vi "Gas Rack Main (FPGA).vi"() -> ()   [LabVIEW 2013]
uses:
  TypeDef/FPGADataCluster.ctl
  <vilib>/Platform/TimedLoop/XDataNode/timing_clust.ctl
  <vilib>/Platform/TimedLoop/XDataNode/nitl_modes.ctl
  <vilib>/Platform/TimedLoop/XDataNode/wakeup.ctl
  <vilib>/rvi/FXPMathLib/basic elements/FxpIntAccumulator/subVIs/nifxpmath_IntAccumulator_SimConfig.ctl
  <vilib>/rvi/FXPMathLib/FxpSqrt/subVIs/nifxpmath_Sqrt_SimConfig.ctl
  <vilib>/fxp/LVFixedPointOverflowPolicyTypeDef.ctl
  <vilib>/rvi/Emulation/niFpgaSctlEmulationGetInTimedLoop.vi
  <vilib>/rvi/Emulation/niFpgaEmulationReportErrorSimple.vi
  <vilib>/rvi/Emulation/niFpgaGetClockAttributes.vi
  <vilib>/rvi/eio/common/nirviEmuTemplateMethod_errors.vi
  <vilib>/rvi/Analysis/common/codeGenErrors/XNode/niFpgaXNodeCodeGenErrorHandle.vi
  <vilib>/rvi/Emulation/niFpgaCriticalErrorInLSC.vi
  <vilib>/rvi/FXPMathLib/basic elements/FxpIntAccumulator/simVIs/DllFxpIntAccumulator_sub.vi
  <vilib>/rvi/interface/RandomDataEmulation/nirviRandomDataFPGAFIFO.vi
  <vilib>/rvi/interface/RandomDataEmulation/niFpgaRandomDataHandleErrors.vi
  <vilib>/rvi/FXPMathLib/FxpSqrt/simVIs/DllSqrtTemp_sub.vi
  <vilib>/rvi/FXPMathLib/FxpSub/XNode/nifxpmath_Sub.xnode
  <vilib>/eio/EIONode/EIONode.xnode
  <vilib>/rvi/Analysis/measure/mean-var-std/XNode/niFpgaMean-Var-Std.xnode
  <vilib>/Platform/TimedLoop/XDataNode/XDataNode.xnode
  <vilib>/rvi/FXPMathLib/basic elements/FxpIntAccumulator/XNode/nifxpmath_IntAccumulator.xnode
  <vilib>/rvi/FXPMathLib/FxpMul/XNode/nifxpmath_Multiplier.xnode
  <vilib>/rvi/DataTransferAndStorage/Container/XNode/niFpgaContainer.xnode
  <vilib>/rvi/interface/RandomDataEmulation/nirviRandomDataFpgaReadWriteTemplate.vi
  <vilib>/rvi/Analysis/measure/butterworth/XNode/niFpgaButterworthFilter.xnode
  <vilib>/rvi/Analysis/measure/dc-rms/XNode/niFpgaDC-RMS.xnode
  <vilib>/rvi/FXPMathLib/FxpSqrt/XNode/nifxpmath_Sqrt.xnode
  <vilib>/Platform/TimedLoop/XDataNode/XDNodeRunTimeDep.lvlib
  <vilib>/rvi/FXPMathLib/sim/FxpSim.dll
panel:
  in  "CtCuttoff":fxp<+,24,5>
  in  "Brushed Speed":bool
  in  "StableTrigger":fxp<+/-,20,5>
  in  "Count 2(uS)":u32=20
  out "AI3":fxp<+/-,24,5>
  out "AI7":fxp<+/-,24,5>
  out "AI6":fxp<+/-,24,5>
  out "AI4":fxp<+/-,24,5>
  out "AI2":fxp<+/-,24,5>
  out "AI1":fxp<+/-,24,5>
  out "AI0":fxp<+/-,24,5>
  out "Actual Loop Time 2":u32
  out "Actual Loop Time":u32
  in  "Count 1(uS)":u32=100
  in  "Hysteresis":fxp<+,24,5>
  out "DataCluster":T1 {"Speed" format="%#_6f"; "Controller Voltage" format="%#_6f"; "Controller Current" format="%#_6f"; "Temperature" format="%#_6f"}
  in  "PWM Period (ticks)":u32
  in  "PWM Duty":i32
  in  "Deadhead":bool
  in  "PSenable":bool
  in  "PresCtrl":fxp<+/-,20,5>
  in  "VoltCtrl":fxp<+/-,20,5>
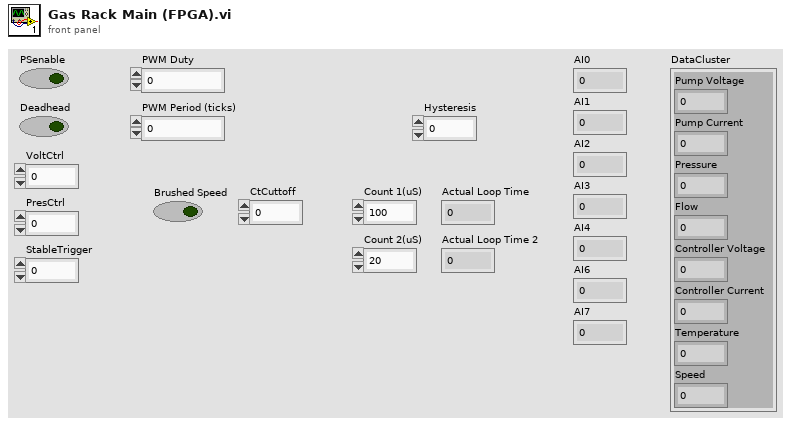
[diagram p1: front panel]
types:
  T1 = typedef "FPGADataCluster.ctl" = cluster{"Pump Voltage":fxp<+/-,25,15>, "Pump Current":fxp<+/-,25,15>, "Pressure":fxp<+/-,25,15>, "Flow":fxp<+/-,25,15>, "Controller Voltage":fxp<+/-,25,15>, "Controller Current":fxp<+/-,25,15>, "Temperature":fxp<+/-,25,15>, "Speed":fxp<+/-,25,15>}
  T2 = typedef "XDNodeRunTimeDep.lvlib/timing_clust.ctl" = cluster{"Expected End [f-1]":u64, "Actual End [f-1]":u64, "Finished Late? [f-1]":bool, "Expected End [i-1]":u64, "Actual End [i-1]":u64, "Finished Late? [i-1]":bool, "Expected Start [i]":u64, "Actual Start [i]":u64, "Expected Start [f]":u64, "Actual Start [f]":u64, "Source Name":string, "Structure Name":string, "Period":i64, "Deadline":i64, "Offset":i64, "Start":i64, "Priority":i32, "Timeout":i32, "Mode":T3, "Wakeup Reason":T4, "Error":errorcluster, "Source Type":string, "Secondary Source Type":string, "Global End Time":u64, "Global Start Time":u64, "Frame Duration":u64, "Iteration Duration":u64, "Assigned CPU":i32, "I/O Scan Engine Mode":u32}
  T3 = typedef "XDNodeRunTimeDep.lvlib/nitl_modes.ctl" = enum32{"No Change", "Process missed periods, maintain original phase", "Discard missed periods, maintain original phase", "Process missed periods, ignore original phase", "Discard missed periods, ignore original phase"}
  T4 = typedef "XDNodeRunTimeDep.lvlib/wakeup.ctl" = enum32{"Normal", "Aborted", "Asynchronous wakeup", "Timing source error", "Timed loop error", "Timeout"}
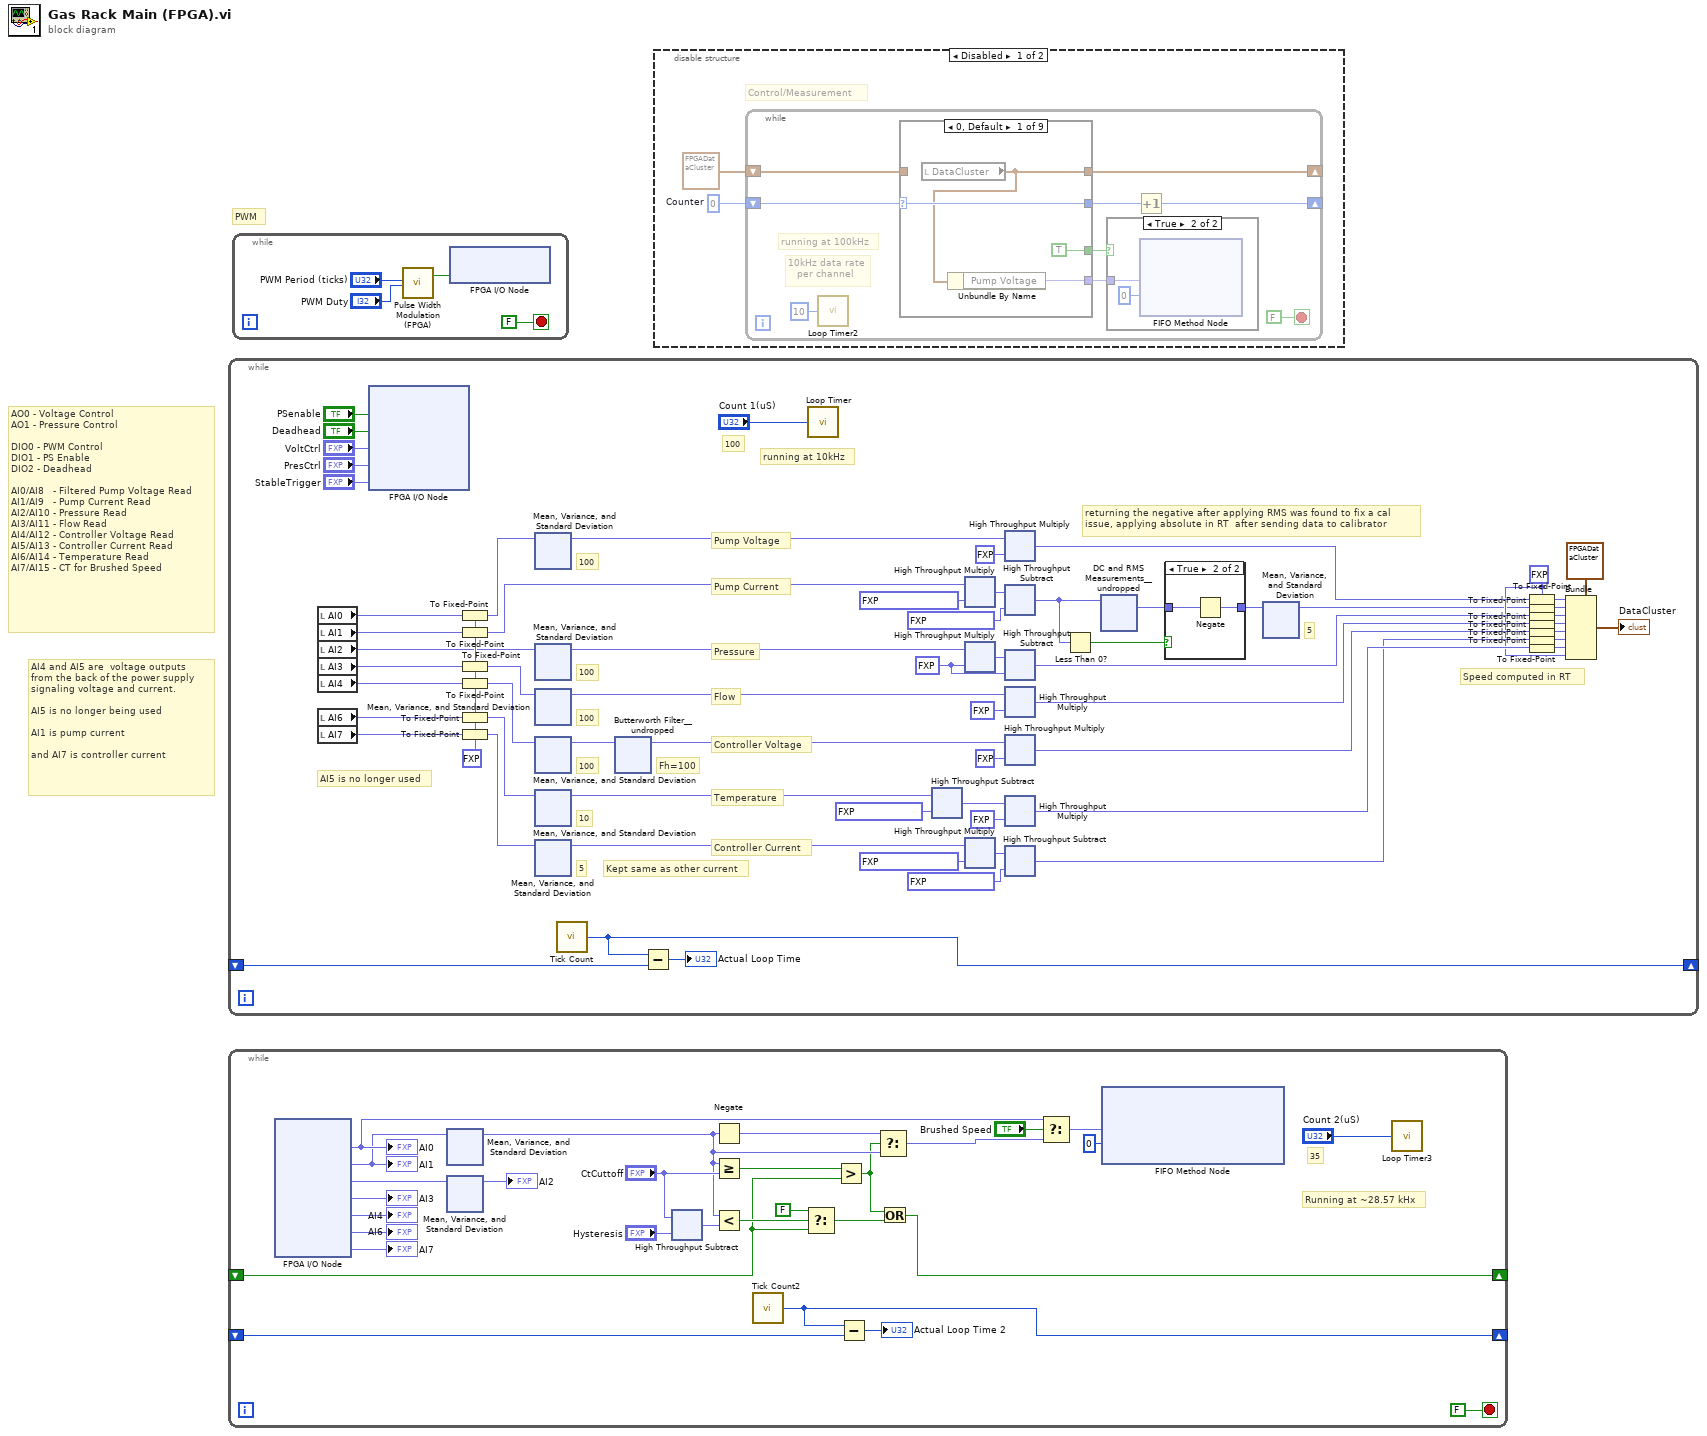
[diagram p0: block diagram]
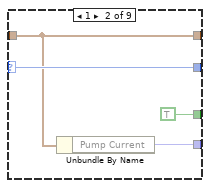
[diagram p3: hidden frame]
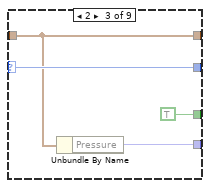
[diagram p4: hidden frame]
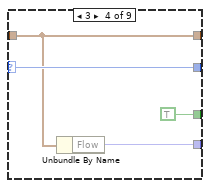
[diagram p5: hidden frame]
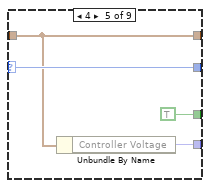
[diagram p6: hidden frame]
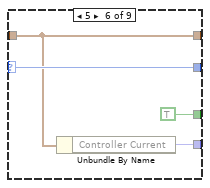
[diagram p7: hidden frame]
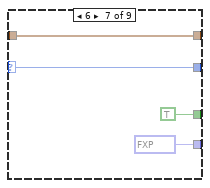
[diagram p8: hidden frame]
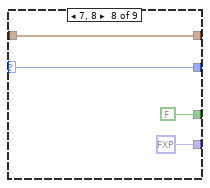
[diagram p9: hidden frame]
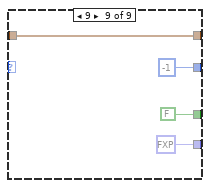
[diagram p10: hidden frame]
diagram:
  # "PWM"
  # "AI4 and AI5 are  voltage outputs\nfrom the back of the power supply\nsignaling voltage and current.\n\nAI5 is no longer being used\n\nAI1 is pump current\n\nand AI7 is controller current"
  # "AO0 - Voltage Control\nAO1 - Pressure Control\n\nDIO0 - PWM Control\nDIO1 - PS Enable\nDIO2 - Deadhead\n\nAI0/AI8   - Filtered Pump Voltage Read\nAI1/AI9   - Pump Current Read\nAI2/AI10 - Pressure Read\nAI3/AI11 - Flow Read\nAI4/AI12 - Controller Voltage Read\nAI5/AI13 - Controller Current Read\nAI6/AI14 - Temperature Read\nAI7/AI15 - CT for Brushed Speed"
  n1 = while {
    shift-right: [w26] -> _
    shift-left: _ -> [w25]
    stop <- FALSE stop-if-true
    w13 = fxp<+,9,9> 350.0 ("y")
    w39 = fxp<+,24,5> 0.0 ("AI4")
    w4 = fxp<+/-,25,15> 0.0 ("Element")
    # "Kept same as other current"
    # "Fh=100"
    # "10"
    # "100"
    # "100"
    # "100"
    # "100"
    # "5"
    # "5"
    # "Temperature"
    # "Controller Current"
    # "Controller Voltage"
    # "Flow"
    # "Pressure"
    # "Pump Current"
    # "Pump Voltage"
    # "100"
    # "Speed computed in RT"
    # "returning the negative after applying RMS was found to fix a cal\nissue, applying absolute in RT  after sending data to calibrator"
    # "AI5 is no longer used"
    # "running at 10kHz"
    n2 = local read "AI0"() -> (w24:fxp<+/-,24,5>)
    n3 = local read "AI1"() -> (w23:fxp<+/-,24,5>)
    n4 = local read "AI2"() -> (w8:fxp<+/-,24,5>)
    n5 = local read "AI3"() -> (w21:fxp<+/-,24,5>)
    n6 = local read "AI4"() -> (w20:fxp<+/-,24,5>)
    n7 = local read "AI6"() -> (w19:fxp<+/-,24,5>)
    n8 = local read "AI7"() -> (w22:fxp<+/-,24,5>)
    n9 = xnode "FPGA I/O Node"("RMC/DIO1"="PSenable", "RMC/DIO2"="Deadhead", "AO0"="VoltCtrl", "AO1"="PresCtrl", "AO2"="StableTrigger") -> ()  [unwired: 5 in, 5 out]
    n10 = To Fixed-Point(fixed-point type=w39, number=w24) -> (fixed-point=w29:fxp<+,24,5>)
    n11 = To Fixed-Point(fixed-point type=w39, number=w23) -> (fixed-point=w3:fxp<+,24,5>)
    n12 = To Fixed-Point(fixed-point type=w39, number=w21) -> (fixed-point=w38:fxp<+,24,5>)
    n13 = To Fixed-Point(fixed-point type=w39, number=w20) -> (fixed-point=w37:fxp<+,24,5>)
    n14 = To Fixed-Point(fixed-point type=w39, number=w19) -> (fixed-point=w28:fxp<+,24,5>)
    n15 = To Fixed-Point(fixed-point type=w39, number=w22) -> (fixed-point=w10:fxp<+,24,5>)
    n16 = xnode "Mean, Variance, and Standard Deviation"("input data"=w29) -> ("mean"=w36:fxp<+,24,5>)  [unwired: 1 in, 1 out]
    n17 = xnode "Mean, Variance, and Standard Deviation"("input data"=w8) -> ("mean"=w7:fxp<+/-,24,5>)  [unwired: 1 in, 1 out]
    n18 = xnode "Mean, Variance, and Standard Deviation"("input data"=w38) -> ("mean"=w35:fxp<+,24,5>)  [unwired: 1 in, 1 out]
    n19 = xnode "Mean, Variance, and Standard Deviation"("input data"=w37) -> ("mean"=w6:fxp<+,24,5>)  [unwired: 1 in, 1 out]
    n20 = xnode "Mean, Variance, and Standard Deviation"("input data"=w28) -> ("mean"=w33:fxp<+,24,5>)  [unwired: 1 in, 1 out]
    n21 = xnode "Mean, Variance, and Standard Deviation"("input data"=w10) -> ("mean"=w9:fxp<+,24,5>)  [unwired: 1 in, 1 out]
    n22 = call "Tick Count"() -> ("Tick Count(uSec)"=w26:u32)
    n23 = xnode "Butterworth Filter__undropped"("input data"=w6) -> ("output data"=w5:fxp<+/-,29,10>)  [unwired: 2 in]
    n24 = Subtract(x=w26, y=w25) -> (x-y=→"Actual Loop Time":u32)
    n25 = call "Loop Timer"("Count(uSec)"="Count 1(uS)") -> ()  [unwired: 1 out]
    n26 = xnode "High Throughput Subtract"("x"=w33, "y"=fxp<+/-,20,7> 3.300048828125) -> ("x-y"=w32:fxp<+/-,21,10>)
    n27 = xnode ("High Throughput Multiply")("x"=w3, "y"=fxp<+/-,20,7> 24.0384521484375 ("Volt")) -> ("x*y"=w64:fxp<+/-,44,12>)
    n28 = xnode ("High Throughput Multiply")("x"=w7, "y"=w13) -> ("x*y"=w15:fxp<+/-,33,14>)
    n29 = xnode ("High Throughput Multiply")("x"=w9, "y"=fxp<+/-,20,7> 24.0384521484375 ("Volt")) -> ("x*y"=w30:fxp<+/-,44,12>)
    n30 = xnode ("High Throughput Multiply")("x"=w36, "y"=fxp<+/-,24,5> 11.0) -> ("x*y"=w45:fxp<+/-,25,15>)
    n31 = xnode "High Throughput Subtract"("x"=w64, "y"=fxp<+/-,20,7> 60.09619140625 ("Volt")) -> ("x-y"=w12:fxp<+/-,25,15>)
    n32 = xnode "High Throughput Subtract"("x"=w15, "y"=w13) -> ("x-y"=w14:fxp<+/-,34,15>)
    n33 = xnode ("High Throughput Multiply")("x"=w35, "y"=fxp<+,8,8> 210.0) -> ("x*y"=w44:fxp<+/-,25,15>)
    n34 = xnode ("High Throughput Multiply")("x"=w5, "y"=fxp<+,8,8> 11.0) -> ("x*y"=w43:fxp<+/-,25,15>)
    n35 = xnode ("High Throughput Multiply")("x"=w32, "y"=fxp<+/-,9,9> 200.0) -> ("x*y"=w31:fxp<+/-,25,15>)
    n36 = xnode "High Throughput Subtract"("x"=w30, "y"=fxp<+/-,20,7> 60.09619140625 ("Volt")) -> ("x-y"=w11:fxp<+/-,25,15>)
    n37 = Less Than 0?(x=w12) -> (x < 0?=w17:bool)
    n38 = xnode "DC and RMS Measurements__undropped"("input data"=w12) -> ("RMS"=w16:fxp<+,25,15>)  [unwired: 1 in, 1 out]
    n39 = case shown="True" w17 {
      tunnel: w16 -> [w303 w305]
      tunnel: [w303 w304] -> w2
      frame False {
      }
      frame True {
        n40 = Negate(x=w305) -> (-x=w304:fxp<+/-,26,16>)
      }
    }
    n41 = xnode "Mean, Variance, and Standard Deviation"("input data"=w2) -> ("mean"=w1:fxp<+/-,26,16>)  [unwired: 1 in, 1 out]
    n42 = To Fixed-Point(fixed-point type=w4, number=w45) -> (fixed-point=w52:fxp<+/-,25,15>)
    n43 = To Fixed-Point(fixed-point type=w4, number=w1) -> (fixed-point=w53:fxp<+/-,25,15>)
    n44 = To Fixed-Point(fixed-point type=w4, number=w14) -> (fixed-point=w54:fxp<+/-,25,15>)
    n45 = To Fixed-Point(fixed-point type=w4, number=w44) -> (fixed-point=w55:fxp<+/-,25,15>)
    n46 = To Fixed-Point(fixed-point type=w4, number=w43) -> (fixed-point=w56:fxp<+/-,25,15>)
    n47 = To Fixed-Point(fixed-point type=w4, number=w11) -> (fixed-point=w47:fxp<+/-,25,15>)
    n48 = To Fixed-Point(fixed-point type=w4, number=w31) -> (fixed-point=w48:fxp<+/-,25,15>)
    n49 = Bundle(cluster=T1 {"Pump Voltage"=0.0, "Pump Current"=0.0, "Pressure"=0.0, "Flow"=0.0, "Controller Voltage"=0.0, "Controller Current"=0.0, "Temperature"=0.0, "Speed"=0.0} ("DataCluster"), "Pump Voltage"=w52, "Pump Current"=w53, "Pressure"=w54, "Flow"=w55, "Controller Voltage"=w56, "Controller Current"=w47, "Temperature"=w48, "Speed"=w4) -> (→"DataCluster":T1)
  }
  n50 = while {
    shift-right: [w743] -> _
    shift-left: _ -> [w744]
    shift-right: [w720] -> _
    shift-left: _ -> [w724]
    stop <- FALSE stop-if-true
    # "Running at ~28.57 kHx"
    # "35"
    n51 = xnode "FPGA I/O Node"() -> ("AI0"=w733:fxp<+/-,24,5>, "AI1"=w731:fxp<+/-,24,5>, "AI2"=w719:fxp<+/-,24,5>, "AI3"=→"AI3":fxp<+/-,24,5>, "AI4"=→"AI4":fxp<+/-,24,5>, "AI6"=→"AI6":fxp<+/-,24,5>, "AI7"=→"AI7":fxp<+/-,24,5>)  [unwired: 7 in, 7 out]
    "AI0" <- w733
    "AI1" <- w731
    n52 = xnode "Mean, Variance, and Standard Deviation"("input data"=w731) -> ("mean"=w727:fxp<+/-,24,5>)  [unwired: 1 in, 1 out]
    n53 = xnode "Mean, Variance, and Standard Deviation"("input data"=w719) -> ("mean"=→"AI2":fxp<+/-,24,5>)  [unwired: 1 in, 1 out]
    n54 = xnode "High Throughput Subtract"("x"="CtCuttoff", "y"="Hysteresis") -> ("x-y"=w726:fxp<+/-,25,15>)
    n55 = Negate(x=w727) -> (-x=w736:fxp<+/-,25,6>)
    n56 = Greater Or Equal?(x=w727, y="CtCuttoff") -> (x >= y?=w732:bool)
    n57 = Less?(x=w727, y=w726) -> (x < y?=w725:bool)
    n58 = call "Tick Count2"() -> ("Tick Count(uSec)"=w743:u32)
    n59 = Select(t=FALSE, s=w725, f=w724) -> (s? t:f=w722:bool)
    n60 = Greater?(x=w732, y=w724) -> (0:w721:bool)
    n61 = Subtract(x=w743, y=w744) -> (x-y=→"Actual Loop Time 2":u32)
    n62 = Select(t=w736, s=w721, f=w727) -> (s? t:f=w734:fxp<+/-,25,6>)
    n63 = Or(x=w721, y=w722) -> (x .or. y?=w720:bool)
    n64 = Select(t=w733, s="Brushed Speed", f=w734) -> (s? t:f=w730:fxp<+/-,25,6>)
    n65 = xnode ("FIFO Method Node")("Element"=w730, "Timeout"=0) -> ()  [unwired: 1 in, 2 out]
    n66 = call "Loop Timer3"("Count(uSec)"="Count 2(uS)") -> ()  [unwired: 1 out]
  }
  n67 = while {
    stop <- FALSE stop-if-true
    n68 = call "Pulse Width Modulation (FPGA).vi"("PWM Period (Ticks)"="PWM Period (ticks)", "PWM Duty Cycle (Ticks)"="PWM Duty") -> ("PWM DO"=w902:bool)  [unwired: 14 in, 3 out]
    n69 = xnode "FPGA I/O Node"("RMC/DIO0"=w902) -> ()  [unwired: 1 in, 1 out]
  }
  n70 = disable-structure shown="Disabled" {
    frame Disabled {
      w904 = i8 0  # Counter
      # "Control/Measurement"
      n71 = while {
        shift-right: [w906] -> _
        shift-left: T1 {"Pump Voltage"=0.0, "Pump Current"=0.0, "Pressure"=0.0, "Flow"=0.0, "Controller Voltage"=0.0, "Controller Current"=0.0, "Temperature"=0.0, "Speed"=0.0} ("DataCluster") -> [w908]
        shift-right: [w909] -> _
        shift-left: w904 -> [w912]
        stop <- FALSE stop-if-true
        # "10kHz data rate\n   per channel"
        # "running at 100kHz"
        n72 = call "Loop Timer2"("Count(uSec)"=u32 10 ("Count(Ticks)")) -> ()  [unwired: 1 out]
        n73 = case shown="0, Default" w912 {
          selector: w912 -> [w919 w923 w927 w931 w935 w939 w941 w946 _]
          tunnel: [w919 w923 w927 w931 w935 w939 w941 w946 i8 -1 ("Counter")] -> w910
          tunnel: w908 -> [_ w922 w926 w930 w934 w938 w942 w947 w951]
          tunnel: [w917 w921 w925 w929 w933 w937 fxp<+/-,25,15> -16384.0 ("Controller Current") fxp<+/-,25,15> 0.0 ("Controller Current") fxp<+/-,25,15> 0.0 ("Controller Current")] -> w907
          tunnel: [w918 w922 w926 w930 w934 w938 w942 w947 w951] -> w906
          tunnel: [TRUE TRUE TRUE TRUE TRUE TRUE TRUE FALSE FALSE] -> w905
          frame 0, Default {
            n74 = local read "DataCluster"() -> (w918:T1)
            n75 = Unbundle By Name(w918) -> ("Pump Voltage"=w917:fxp<+/-,25,15>)
          }
          frame 1 {
            n76 = Unbundle By Name(w922) -> ("Pump Current"=w921:fxp<+/-,25,15>)
          }
          frame 2 {
            n77 = Unbundle By Name(w926) -> ("Pressure"=w925:fxp<+/-,25,15>)
          }
          frame 3 {
            n78 = Unbundle By Name(w930) -> ("Flow"=w929:fxp<+/-,25,15>)
          }
          frame 4 {
            n79 = Unbundle By Name(w934) -> ("Controller Voltage"=w933:fxp<+/-,25,15>)
          }
          frame 5 {
            n80 = Unbundle By Name(w938) -> ("Controller Current"=w937:fxp<+/-,25,15>)
          }
          frame 6 {
          }
          frame 7, 8 {
          }
          frame 9 {
          }
        }
        n81 = case shown="True" w905 {
          tunnel: w907 -> [_ w915]
          frame False {
          }
          frame True {
            n82 = xnode ("FIFO Method Node")("Element"=w915, "Timeout"=0) -> ()  [unwired: 1 in, 2 out]
          }
        }
        n83 = Increment(x=w910) -> (x+1=w909:i8)
      }
    }
    frame Enabled {
    }
  }
